vi "LJcounterUD_Debounce.vi"() -> ()   [LabVIEW 2021]
panel:
  in  "Write On Change":bool
  in  "Data File":path=path "c:/temp/data.dat"
  in  "Write To File":bool
  in  "Reset Counter":bool=TRUE
  in  "Measurement Type":u16(ring) items=["Frequency", "Count"]
  out "Measurement":dbl format="%.2f"
  out "Error Message":string
  in  "stop":bool
  in  "Interval (seconds)":dbl=1.0 min=0.025 format="%.2f"
  # "www.labjack.com"
  # "Uses the first found U3 or UE9 over USB.  Counter appears on FIO0 on the UE9, and\nFIO4 on the U3.  Uses a timer set to mode 6 (Firmware Counter with Debounce).  The\ndefault debounce value is 1, which corresponds to about 87-174 ms on the UE9\nand about 16-32 ms on the U3."
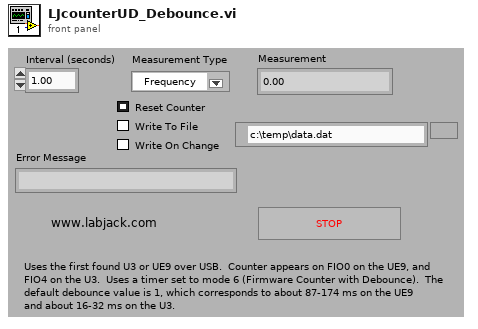
[diagram p1: front panel]
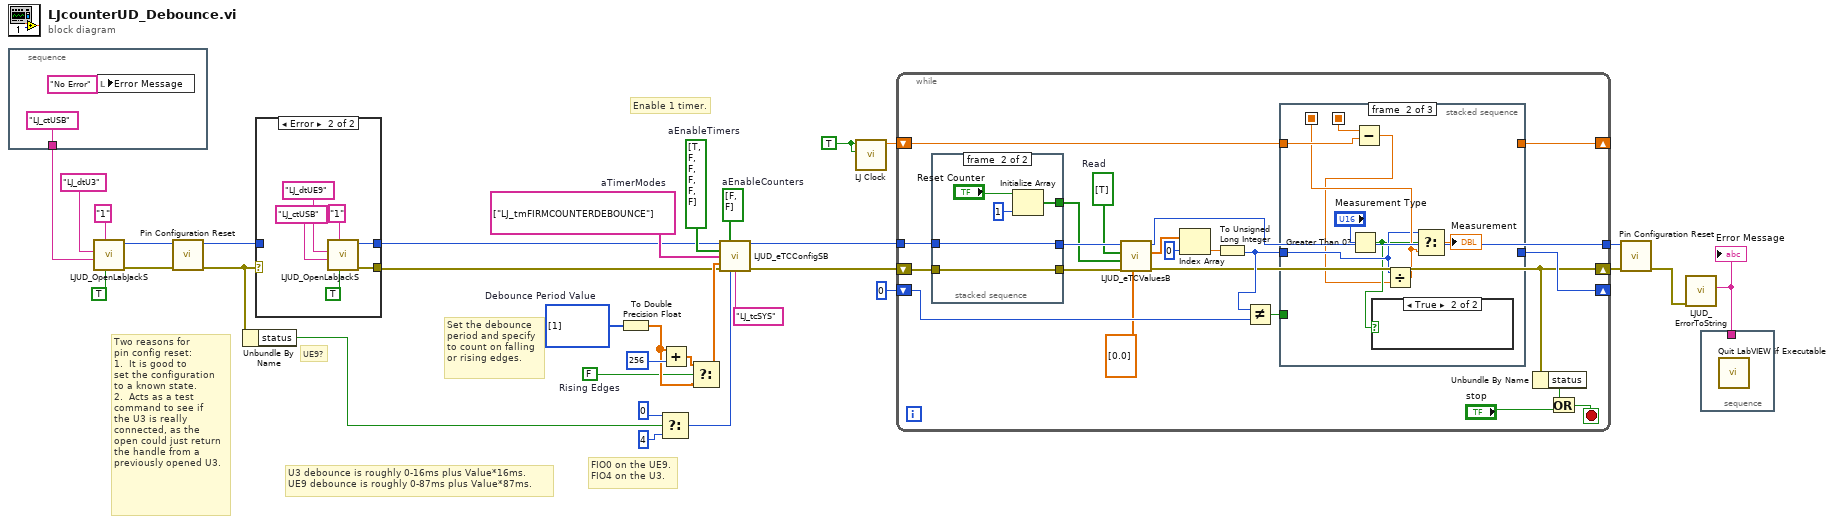
[diagram p0: block diagram]
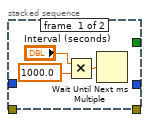
[diagram p2: hidden frame]
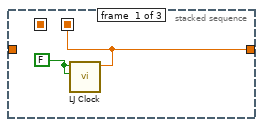
[diagram p3: hidden frame]
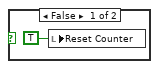
[diagram p4: hidden frame]
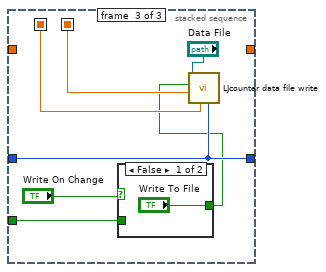
[diagram p5: hidden frame]
diagram:
  w20 = u8[] [1]  # Debounce Period Value
  w21 = FALSE  # Rising Edges
  w24 = bool[] [FALSE, FALSE]  # aEnableCounters
  w25 = bool[] [TRUE, FALSE, FALSE, FALSE, FALSE, FALSE]  # aEnableTimers
  w26 = string[] ["LJ_tmFIRMCOUNTERDEBOUNCE"]  # aTimerModes
  w33 = TRUE ("Initialize")
  # "U3 debounce is roughly 0-16ms plus Value*16ms.\nUE9 debounce is roughly 0-87ms plus Value*87ms."
  # "FIO0 on the UE9.\nFIO4 on the U3."
  # "Two reasons for\npin config reset:\n1.  It is good to\nset the configuration\nto a known state.\n2.  Acts as a test\ncommand to see if\nthe U3 is really\nconnected, as the\nopen could just return\nthe handle from a\npreviously opened U3."
  # "UE9?"
  # "Enable 1 timer."
  # "Set the debounce\nperiod and specify\nto count on falling\nor rising edges."
  n1 = stacked-sequence {
    tunnel: ["LJ_ctUSB" ("ConnectionType")] -> w14
    frame #0 {
      n2 = local write "Error Message"("No Error" ("Error Message")) -> ()
    }
  }
  n3 = call "LJUD_OpenLabJackS.vi"("FirstFound"=TRUE, "Address"="1", "ConnectionType"=w14, "DeviceType"="LJ_dtU3") -> ("error out"=w10:errorcluster, "Handle"=w11:i32)  [unwired: 5 in, 1 out]
  n4 = call "Pin Configuration Reset.vi"("error in"=w10, "Handle In"=w11) -> ("error out"=w9:errorcluster, "Handle Out"=w8:i32)  [unwired: 8 in]
  n5 = Unbundle By Name(w9) -> ("status"=w3:bool)
  n6 = case shown="Error" w9 {
    selector: w9 -> [w36 _]
    tunnel: [w36 w39] -> w6
    tunnel: [w37 w38] -> w7
    tunnel: w8 -> [w37 _]
    frame No Error {
    }
    frame Error {
      n7 = call "LJUD_OpenLabJackS.vi"("FirstFound"=TRUE, "Address"="1", "ConnectionType"="LJ_ctUSB", "DeviceType"="LJ_dtUE9") -> ("error out"=w39:errorcluster, "Handle"=w38:i32)  [unwired: 5 in, 1 out]
    }
  }
  n8 = To Double Precision Float(number=w20) -> (double precision float=w28:dbl[])
  n9 = Select(t=0 ("TCPinOffset"), s=w3, f=4) -> (s? t:f=w4:i32)
  n10 = Add(x=w28, y=256) -> (x+y=w27:dbl[])
  n11 = Select(t=w27, s=w21, f=w28) -> (s? t:f=w30:dbl[])
  n12 = call "LJUD_eTCConfigSB.vi"("Handle In"=w7, "aEnableCounters"=w24, "aEnableTimers"=w25, "aTimerModes"=w26, "aTimerValues"=w30, "error in"=w6, "TCPinOffset"=w4, "TimerClockBase"="LJ_tcSYS") -> ("Handle Out"=w22:i32, "error out"=w23:errorcluster)  [unwired: 6 in]
  n13 = call "LJ Clock.vi"("Sync to second"=w33, "Initialize"=w33) -> ("Seconds since 1/1/1904 universal time"=w32:ext)  [unwired: 9 in]
  n14 = while {
    tunnel: [w48] -> w16
    tunnel: w22 -> [w57]
    shift-left: w23 -> [w60]
    shift-right: [w52] -> w18
    shift-left: u32 0 -> [w53]
    shift-right: [w61] -> _
    shift-left: w32 -> [w63]
    shift-right: [w64] -> _
    stop <- w49 stop-if-true
    w47 = bool[] [TRUE]  # Read
    n15 = stacked-sequence {
      tunnel: w60 -> [_ w72]
      tunnel: [_ w72] -> w59
      tunnel: [_ w71] -> w58
      tunnel: w57 -> [_ w71]
      tunnel: [_ w68] -> w46
      frame #0 {
        n16 = Multiply(x="Interval (seconds)", y=1000.0) -> (x*y=w66:dbl)
        n17 = Wait Until Next ms Multiple(millisecond multiple=w66) -> ()  [unwired: 1 out]
      }
      frame #1 {
        n18 = Initialize Array("Reset Counter", 1 ("Dimension Size")) -> (w68:bool[])
      }
    }
    n19 = call "LJUD_eTCValuesB.vi"("aTimerValues Write"=dbl[] [0.0], "error in"=w59, "aUpdateResetTimers"=w46, "aReadTimers"=w47, "Handle In"=w58) -> ("error out"=w52:errorcluster, "aTimerValues Read"=w44:dbl[], "Handle Out"=w48:i32)  [unwired: 3 in, 1 out]
    n20 = Index Array(array=w44, index=0 ("Index")) -> (element=w55:dbl)
    n21 = To Unsigned Long Integer(number=w55) -> (unsigned 32bit integer=w54:u32)
    n22 = Not Equal?(x=w54, y=w53) -> (x != y?=w62:bool)
    n23 = stacked-sequence {
      seq-local: [w73 _ _] -> [_ w80 w89]
      seq-local: [_ w78 _] -> [_ _ w88]
      tunnel: w54 -> [_ w77 w85]
      tunnel: [w73 _ _] -> w64
      tunnel: w63 -> [_ w79 _]
      tunnel: w62 -> [_ _ w86]
      tunnel: [_ _ w85] -> w61
      frame #0 {
        w74 = FALSE ("Initialize")
        n24 = call "LJ Clock.vi"("Sync to second"=w74, "Initialize"=w74) -> ("Seconds since 1/1/1904 universal time"=w73:ext)  [unwired: 9 in]
      }
      frame #1 {
        n25 = Greater Than 0?(x="Measurement Type") -> (x > 0?=w76:bool)
        n26 = Subtract(x=w80, y=w79) -> (x-y=w75:ext)
        n27 = case shown="True" w76 {
          frame False {
            n28 = local write "Reset Counter"(TRUE ("Reset Counter")) -> ()
          }
          frame True {
          }
        }
        n29 = Divide(x=w77, y=w75) -> (x/y=w78:ext)
        n30 = Select(t=w77, s=w76, f=w78) -> (s? t:f=→"Measurement":ext)
      }
      frame #2 {
        n31 = case shown="False" "Write On Change" {
          tunnel: w86 -> [_ w92]
          tunnel: ["Write To File" w92] -> w84
          frame False {
          }
          frame True {
          }
        }
        n32 = call "LJcounter data file write.vi"("Count"=w85, "Frequency"=w88, "seconds"=w89, "Write To File"=w84, "Data File"="Data File") -> ()  [unwired: 6 in, 1 out]
      }
    }
    n33 = Unbundle By Name(w52) -> ("status"=w51:bool)
    n34 = Or(x=w51, y="stop") -> (x .or. y?=w49:bool)
  }
  n35 = call "Pin Configuration Reset.vi"("error in"=w18, "Handle In"=w16) -> ("error out"=w19:errorcluster)  [unwired: 8 in, 1 out]
  n36 = call "LJUD_ErrorToString.vi"("error in"=w19) -> ("String"=w17:string)  [unwired: 10 in]
  "Error Message" <- w17
  n37 = stacked-sequence {
    tunnel: w17 -> [_]
    frame #0 {
      n38 = call "Quit LabVIEW if Executable.vi"() -> ()  [unwired: 1 in]
    }
  }
